vi ".NET Type Builder Define Assembly.vi"(8 "error in (no error)":errorcluster, 9 "Access (Run and Collect)":i32(ring)=9 items=["Run"=1, "Save"=2, "Run and Save"=3, "Reflection Only"=6, "Run and Collect"=9], 10 "Name":string) -> (0 "error out":errorcluster, 1 ".NET Assembly Builder":refnum<k24>)   [LabVIEW 2018, in "TwinCAT ADS.lvclass"]
uses:
  TwinCAT ADS.lvclass
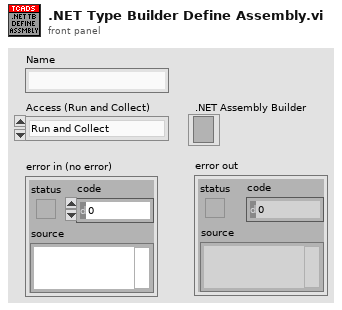
[diagram p1: front panel]
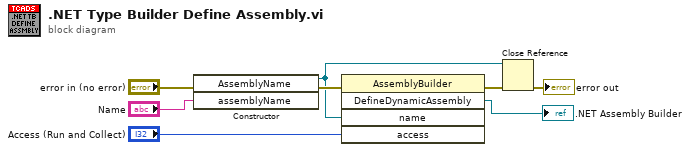
[diagram p0: block diagram]
diagram:
  n1 = constructor class="AssemblyName"(error in="error in (no error)", "assemblyName"="Name") -> (reference out=w2:refnum<k24>, error out=w8:errorcluster)  [unwired: 2 in, 2 out]
  n2 = invoke class="AssemblyBuilder" method="DefineDynamicAssembly"(error in=w8, "name"=w2, "access"="Access (Run and Collect)") -> (error out=w4:errorcluster, "DefineDynamicAssembly"=→".NET Assembly Builder":refnum<k24>)  [unwired: 2 in, 3 out]
  n3 = Close Reference(reference=w2, error in (no error)=w4) -> (error out=→"error out":errorcluster)
